vi "Write Signal Ref.vi"(8 "error in (no error)":errorcluster, 10 "Signal Ref":refnum<vi>, 11 "Data Saver in":refnum<class "Data Saver.lvclass">) -> (0 "error out":errorcluster, 3 "Data Saver out":refnum<class "Data Saver.lvclass">)   [LabVIEW 2014, in "Data Saving.lvlib" / "Data Saver.lvclass"]
uses:
  Data Saver.lvclass
  Data Saver.lvclass/Data Saver.ctl
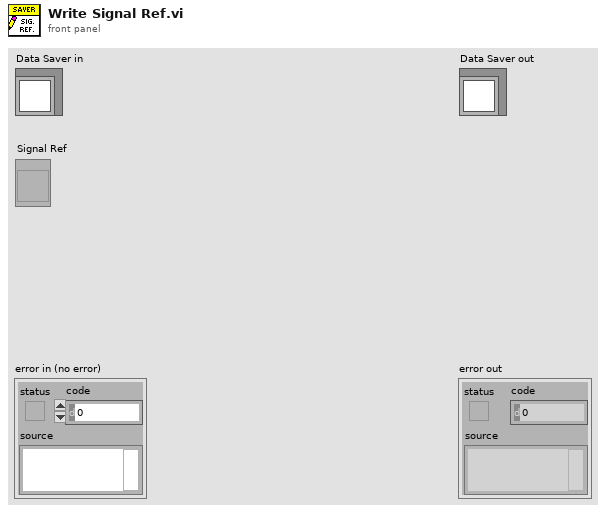
[diagram p1: front panel]
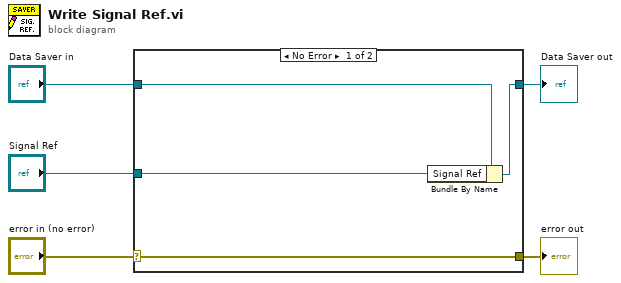
[diagram p0: block diagram]
diagram:
  n1 = case shown="No Error" "error in (no error)" {
    selector: "error in (no error)" -> [w9 w10]
    tunnel: [w9 w10] -> w4
    tunnel: [w7 w11] -> w2
    tunnel: "Data Saver in" -> [w8 w11]
    tunnel: "Signal Ref" -> [w6 _]
    frame No Error {
      n2 = Bundle By Name(cluster=w8, "Signal Ref"=w6) -> (w7:refnum<class "Data Saver.lvclass">)
    }
    frame Error {
    }
  }
  "error out" <- w4
  "Data Saver out" <- w2
